vi "memory_test.vi"() -> ()   [LabVIEW 2009]
uses:
  <vilib>/rvi/LocalResourceManager/LocalResourceManager.xnode
  <vilib>/rvi/eio/common/nirviEmuReportErrorAndStop.vi
  <vilib>/rvi/DataTransferAndStorage/Container/Common/niFpgaContainerSetEmuInfo.vi
  <vilib>/rvi/DataTransferAndStorage/Container/Common/niFpgaContainerState.ctl
  <vilib>/rvi/DataTransferAndStorage/Container/Common/niFpgaDataTypeControl.ctl
  <vilib>/rvi/DataTransferAndStorage/Container/Common/niFpgaContainerImplementationControl.ctl
  <vilib>/rvi/DataTransferAndStorage/Container/Common/niFpgaContainerArbitrationOptionsControl.ctl
  <vilib>/rvi/DataTransferAndStorage/Container/Common/niFpgaTransferTypeControl.ctl
  <vilib>/rvi/DataTransferAndStorage/Container/Common/niFpgaContainerInitializationParameters.ctl
  <vilib>/rvi/DataTransferAndStorage/Container/Common/niFpgaContainerMetaDataKey.ctl
panel:
  out "Array Element":u8
  in  "New element":u8
  out "Time 2":u32
  out "Time":u32
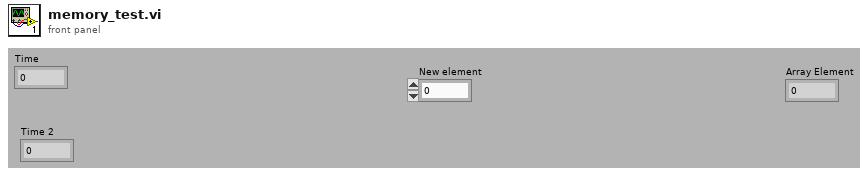
[diagram p1: front panel]
types:
  T1 = typedef "occupancy grid memory typedef.ctl" = refnum<k21>
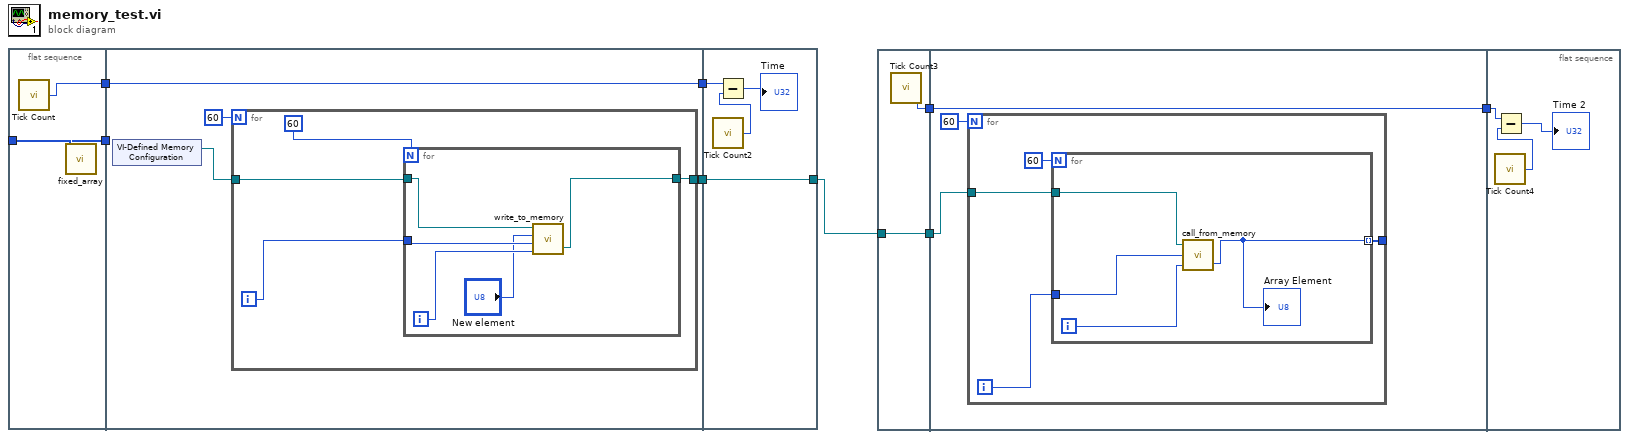
[diagram p0: block diagram]
diagram:
  n1 = flat-sequence {
    tunnel: w4 -> [w11]
    tunnel: [w11] -> w9
    tunnel: [w10] -> w8
    tunnel: w9 -> [_]
    tunnel: w8 -> [w14]
    tunnel: [w14] -> w7
    tunnel: [w13] -> w3
    tunnel: w7 -> [w59]
    tunnel: [w57] -> w1
    tunnel: w3 -> [w57]
    frame #0 {
      n2 = call "Tick Count"() -> ("Tick Count(Ticks)"=w10:u32)
    }
    frame #1 {
      n3 = xnode "VI-Defined Memory Configuration"() -> ("Memory Out"=w12:refnum<k21>)
      n4 = for {
        N: 60 -> [_]
        tunnel: w12 -> [w49]
        tunnel: [w50] -> w13
        i -> [w48]
        n5 = for {
          N: 60 -> [_]
          tunnel: w48 -> [w55]
          tunnel: w49 -> [w56]
          tunnel: [w53] -> w50
          i -> [w54]
          n6 = call "write_to_memory.vi"("Column"=w54, "Row"=w55, "New element"="New element", "Memory Out"=w56) -> ("Memory Out 2"=w53:T1)  [unwired: 1 in]
        }
      }
    }
    frame #2 {
      n7 = call "Tick Count2"() -> ("Tick Count(Ticks)"=w60:u32)
      n8 = Subtract(x=w59, y=w60) -> (x-y=→"Time":u32)
    }
  }
  n9 = call "fixed_array.vi"() -> ("Array"=w4:u8[])  [unwired: 11 in]
  n10 = flat-sequence {
    tunnel: [w62] -> w6
    tunnel: [w61] -> w2
    tunnel: w1 -> [w61]
    tunnel: w6 -> [w64]
    tunnel: [w64] -> w5
    tunnel: w2 -> [w63]
    tunnel: w5 -> [w74]
    frame #0 {
      n11 = call "Tick Count3"() -> ("Tick Count(Ticks)"=w62:u32)
    }
    frame #1 {
      n12 = for {
        N: 60 -> [_]
        tunnel: w63 -> [w67]
        tunnel: [w66] -> _
        i -> [w68]
        n13 = for {
          N: 60 -> [_]
          tunnel: w68 -> [w72]
          tunnel: w67 -> [w71]
          tunnel: [w70] -> w66 mode=indexing
          i -> [w73]
          n14 = call "call_from_memory.vi"("Column"=w73, "Row"=w72, "Memory"=w71) -> ("Array Element"=w70:u8)  [unwired: 1 out]
          "Array Element" <- w70
        }
      }
    }
    frame #2 {
      n15 = call "Tick Count4"() -> ("Tick Count(Ticks)"=w76:u32)
      n16 = Subtract(x=w74, y=w76) -> (x-y=→"Time 2":u32)
    }
  }
